vi "FPGA_InterruptWriteConfiguration.vi"(6 "Falling Edge":bool, 7 "WaitForAck":bool, 8 "error in (no error)":errorcluster, 9 "Rising Edge":bool, 10 "Source":T1={"DevStatus"={"status"=FALSE, "code"=0, "source"=""}, "AnalogTriggerMode?"=FALSE, "DigitalMode"={"DIO Channel"=enum."Disabled"}, "AnalogTriggerMode"={"AnalogTriggerIndex"=enum."Trig 0", "OutputType"=enum."InWindow"}}, 11 "InteruptRef in":T5) -> (0 "error out":errorcluster, 3 "InteruptRef out":T5)   [LabVIEW 2017]
uses:
  <vilib>/Rock Robotics/SystemInterfaces/Interrupt/FPGA_InterruptRef.ctl
  <vilib>/Rock Robotics/SystemInterfaces/Interrupt/FPGA_InterruptIndex.ctl
  <vilib>/Rock Robotics/SystemInterfaces/CounterEncoderSourceConvertion/FPGA_CounterEncoderSourceConvertionLVSourceType.ctl
  <vilib>/Rock Robotics/SystemInterfaces/DIO/FPGA_DIODigitalSourceChannel.ctl
  <vilib>/Rock Robotics/SystemInterfaces/AnalogTrigger/FPGA_AnalogTriggerIndex.ctl
  <vilib>/Rock Robotics/SystemInterfaces/AnalogTrigger/FPGA_AnalogTriggerOutType.ctl
  <vilib>/rvi/errors/niLvFpgaAdjustHostInterfaceError.vi
  <vilib>/Utility/error.llb/Error Cluster From Error Code.vi
  <vilib>/Rock Robotics/SystemInterfaces/System/FPGA_SystemFPGA Ref Global.vi
  <vilib>/Rock Robotics/SystemInterfaces/System/FPGA_SystemFRC FPGA Ref.ctl
  <vilib>/rvi/interface/nirviReadWriteControl/nirviReadWriteControl.xnode
  NiFpgaLv.dll
  <vilib>/rvi/interface/Simulation/niFpgaSimulationCallBeginRW.vi
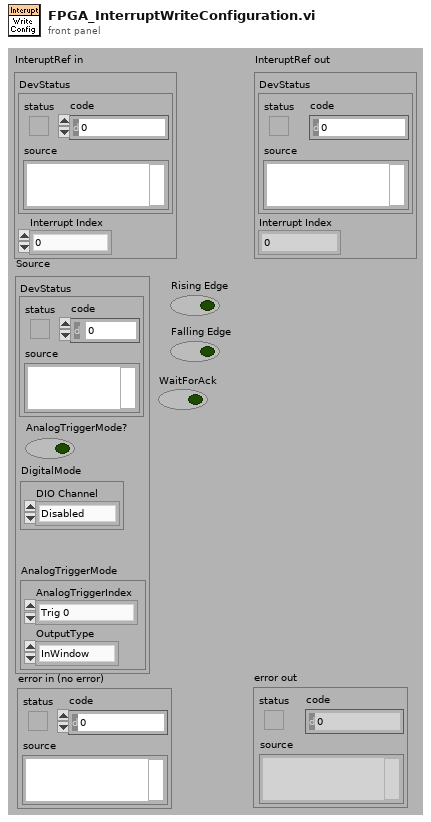
[diagram p1: front panel]
types:
  T1 = typedef "FPGA_CounterEncoderSourceConvertionLVSourceType.ctl" = cluster{"DevStatus":errorcluster, "AnalogTriggerMode?":bool, "DigitalMode":cluster{"DIO Channel":T2}, "AnalogTriggerMode":cluster{"AnalogTriggerIndex":T3, "OutputType":T4}}
  T2 = typedef "FPGA_DIODigitalSourceChannel.ctl" = enum8{"DIO 0", "DIO 1", "DIO 2", "DIO 3", "DIO 4", "DIO 5", "DIO 6", "DIO 7", "DIO 8", "DIO 9", "DIO MXP 0", "DIO MXP 1", "DIO MXP 2", "DIO MXP 3", "DIO MXP 4", "DIO MXP 5", "DIO MXP 6", "DIO MXP 7", "DIO MXP 8", "DIO MXP 9", "DIO MXP 10", "DIO MXP 11", "DIO MXP 12", "DIO MXP 13", "DIO MXP 14", "DIO MXP 15", "Disabled"}
  T3 = typedef "FPGA_AnalogTriggerIndex.ctl" = enum8{"Trig 0", "Trig 1", "Trig 2", "Trig 3", "Trig 4", "Trig 5", "Trig 6", "Trig 7", "Invalid"}
  T4 = typedef "FPGA_AnalogTriggerOutType.ctl" = enum16{"InWindow", "TriggerState", "Rising", "Falling"}
  T5 = typedef "FPGA_InterruptRef.ctl" = cluster{"DevStatus":errorcluster, "Interrupt Index":T6}
  T6 = typedef "FPGA_InterruptIndex.ctl" = enum8{"0", "1", "2", "3", "4", "5", "6", "7", "Invalid"}
  T7 = cluster{"Source":cluster{"Channel":fxp<+,4,4>, "Module":fxp<+,1,1>, "AnalogTrigger":bool}, "RisingEdge":bool, "FallingEdge":bool, "WaitForAck":bool}
  T8 = typedef "FPGA_SystemFRC FPGA Ref.ctl" = refnum<k20>
  T9 = cluster{"Channel":fxp<+,4,4>, "Module":fxp<+,1,1>, "AnalogTrigger":bool}
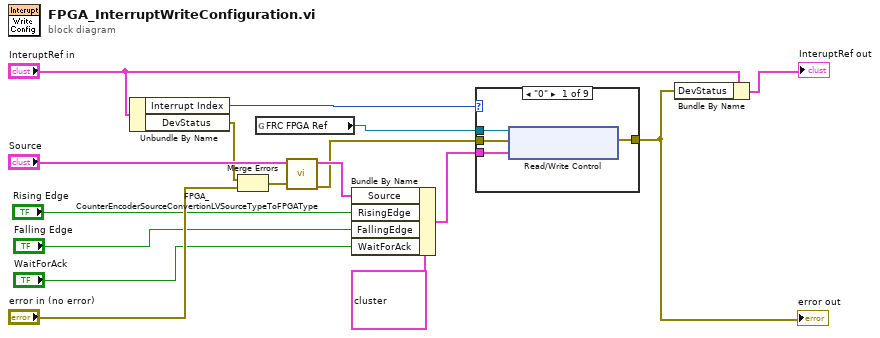
[diagram p0: block diagram]
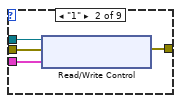
[diagram p2: hidden frame]
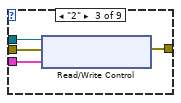
[diagram p3: hidden frame]
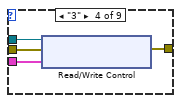
[diagram p4: hidden frame]
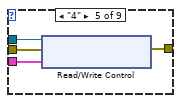
[diagram p5: hidden frame]
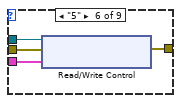
[diagram p6: hidden frame]
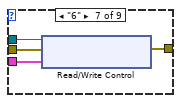
[diagram p7: hidden frame]
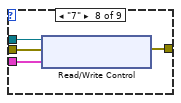
[diagram p8: hidden frame]
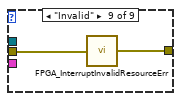
[diagram p9: hidden frame]
diagram:
  n1 = Unbundle By Name("InteruptRef in") -> ("Interrupt Index"=w8:T6, "DevStatus"=w1:errorcluster)
  n2 = Merge Errors(w1, "error in (no error)") -> (w2:errorcluster)
  n3 = global read "FPGA_SystemFPGA Ref Global.vi" "FRC FPGA Ref"() -> (w3:T8)
  n4 = call <vilib>:"FPGA_CounterEncoderSourceConvertionLVSourceTypeToFPGAType.vi"("error in (no error)"=w2, "DigitalSource"="Source") -> ("error out"=w4:errorcluster, "FPGASource"=w7:T9)  [unwired: 8 out]
  n5 = Bundle By Name(cluster=T7 {"Source"={"Channel"=0.0, "Module"=0.0, "AnalogTrigger"=FALSE}, "RisingEdge"=TRUE, "FallingEdge"=FALSE, "WaitForAck"=FALSE} ("Interrupt0.Config"), "Source"=w7, "RisingEdge"="Rising Edge", "FallingEdge"="Falling Edge", "WaitForAck"="WaitForAck") -> (w5:T7)
  n6 = case shown="\"0\"" w8 {
    tunnel: w3 -> [w19 w24 w28 w32 w36 w40 w44 w48 _]
    tunnel: w4 -> [w20 w23 w27 w31 w35 w39 w43 w47 w49]
    tunnel: [w18 w21 w26 w30 w34 w38 w42 w46 w50] -> w13
    tunnel: w5 -> [w17 w22 w25 w29 w33 w37 w41 w45 _]
    frame "0" {
      n7 = xnode "Read/Write Control"("FPGA VI Reference In"=w19, "error in"=w20, "Interrupt0.Config"=w17) -> ("error out"=w18:errorcluster)  [unwired: 1 out]
    }
    frame "1" {
      n8 = xnode "Read/Write Control"("FPGA VI Reference In"=w24, "error in"=w23, "Interrupt1.Config"=w22) -> ("error out"=w21:errorcluster)  [unwired: 1 out]
    }
    frame "2" {
      n9 = xnode "Read/Write Control"("FPGA VI Reference In"=w28, "error in"=w27, "Interrupt2.Config"=w25) -> ("error out"=w26:errorcluster)  [unwired: 1 out]
    }
    frame "3" {
      n10 = xnode "Read/Write Control"("FPGA VI Reference In"=w32, "error in"=w31, "Interrupt3.Config"=w29) -> ("error out"=w30:errorcluster)  [unwired: 1 out]
    }
    frame "4" {
      n11 = xnode "Read/Write Control"("FPGA VI Reference In"=w36, "error in"=w35, "Interrupt4.Config"=w33) -> ("error out"=w34:errorcluster)  [unwired: 1 out]
    }
    frame "5" {
      n12 = xnode "Read/Write Control"("FPGA VI Reference In"=w40, "error in"=w39, "Interrupt5.Config"=w37) -> ("error out"=w38:errorcluster)  [unwired: 1 out]
    }
    frame "6" {
      n13 = xnode "Read/Write Control"("FPGA VI Reference In"=w44, "error in"=w43, "Interrupt6.Config"=w41) -> ("error out"=w42:errorcluster)  [unwired: 1 out]
    }
    frame "7" {
      n14 = xnode "Read/Write Control"("FPGA VI Reference In"=w48, "error in"=w47, "Interrupt7.Config"=w45) -> ("error out"=w46:errorcluster)  [unwired: 1 out]
    }
    frame "Invalid" {
      n15 = call <vilib>:"FPGA_InterruptInvalidResourceErr.vi"("error in (no error)"=w49) -> ("error out"=w50:errorcluster)
    }
  }
  "error out" <- w13
  n16 = Bundle By Name(cluster="InteruptRef in", "DevStatus"=w13) -> (→"InteruptRef out":T5)
